vi "Parse RSB Spoof Telemetry.vi"(11 "Variant_in":variant) -> (3 "FullTelemetry":T1(array[cluster]) {"TelemetryData" format="%04x"; "CommandWord" format="%04x"})   [LabVIEW 2019]
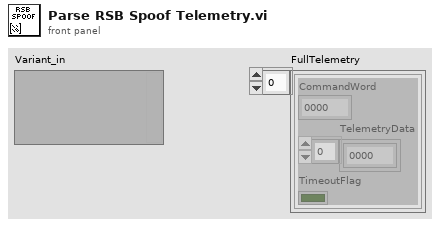
[diagram p1: front panel]
types:
  T1 = cluster{"CommandWord":u16, "TelemetryData":u16[], "TimeoutFlag":bool}[]
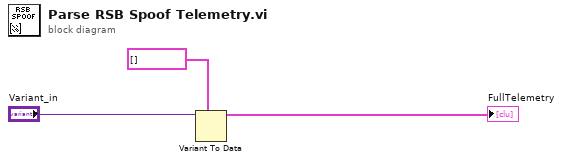
[diagram p0: block diagram]
diagram:
  n1 = Variant To Data(type=T1 [], Variant="Variant_in") -> (data=→"FullTelemetry":T1)  [unwired: 1 in, 1 out]
